vi "NF87XX.get channel.vi"(0 "i ref in":refnum<vi>, 2 "System":string, 5 "error in (no error)":errorcluster) -> (14 "i ref out":refnum<vi>, 16 "Channel":i32, 19 "error out":errorcluster)   [LabVIEW 2014, in "NF87XX.lvlib"]
doc: "Returns the actice motor channel if \"System\" is the name of one of the drivers, the driver is of type 1 (3-channel open loop driver), and the system answers without error. Otherwise 99999 is given out.\n\nauthor: Stefan Götte\ndata: 09-JAN-2007\n\n\nLicense Agreement for this software:\n\nCopyright (C)\nGesellschaft für Schwerionenforschung, GSI\nPlanckstr. 1\n64291 Darmstadt\nGermany\n\nContact: D.Beck@gsi.de \n\nThis program is free software; you can redistribute it and/or modify it under the terms of the GNU General Public License as published by the Free Software Foundation; either version 2 of the license, or (at your option) any later version.\n\nThis program is distributed in the hope that it will be useful, but WITHOUT ANY WARRANTY; without even the implied warranty of MERCHANTABILITY or FITNESS FOR A PARTICULAR PURPOSE. See the GNU General License for more details (http://www.gnu.org).\n\nGesellschaft für Schwerionenforschung, GSI\nPlanckstr. 1, 64291 Darmstadt, Germany\nFor all questions and ideas contact: M.Richter@gsi.de, H.Brand@gsi.de or D.Beck@gsi.de.\nLast update: 17-JUN-2004"
uses:
  NF87XX.lvlib
  instr.lib/NewFocusPico/Pico Parameters.ctl
  instr.lib/NewFocusPico/NewFocusPico - Driver np.lvlib
panel:
  in  "Pico Parameters":T1={"Pico Type"=enum."Open-Loop Pico", "Acceleration (steps/sec^2)"="32000", "Velocity ( Hz)"="2000", "Driver"="A1", "Motor"="0", "Channel"="0", "Process Step"="Final Test"}
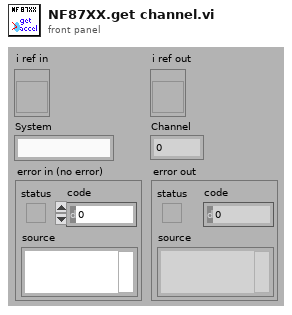
[diagram p1: front panel]
types:
  T1 = typedef "NewFocusPico - Driver np.lvlib/Pico Parameters.ctl" = cluster{"Pico Type":enum16{"Open-Loop Pico", "Close-Loop Pico", "Pico Ultra"}, "Acceleration (steps/sec^2)":string, "Velocity ( Hz)":string, "Driver":string, "Motor":string, "Channel":string, "Process Step":string}
  T2 = typedef "NF87XX.lvlib/NF87XX.driver Type.ctl" = enum16{"not defined", "3-ch open loop drv", "1-ch closed loop drv"}
  T3 = enum16{"User....", "DEF", "DIAG", "INI", "LOCK", "UNLOCK", "MAP", "SAV", "VER", "ACC", "CHL", "FOR", "GO", "HAL", "MOF", "MON", "MPV", "POS", "REL", "REV", "STA", "STO", "TYP", "VEL", "ABS", "SER", "NOS", "DRT", "FLI", "RLI", "FIN", "RIN", "AIN", "IN", "JOF", "JON", "OUT", "RES FINE", "RES COARSE", "02 (HEX)", "PWM", "CNT", "TMR", "HOSTNAME", "IPADDR", "IPMODE", "NETMASK", "GATEWAY", "DNSSRVR", "PASSWD", "ECHO", "MACADDR"}
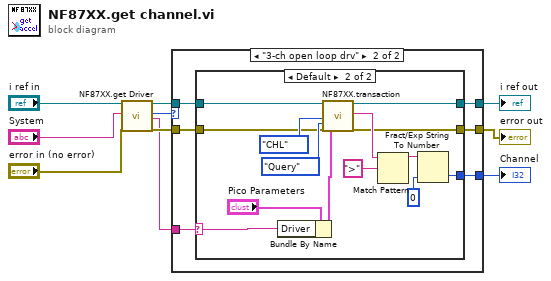
[diagram p0: block diagram]
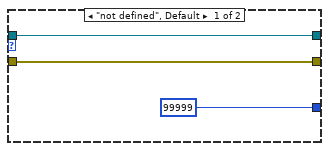
[diagram p2: hidden frame]
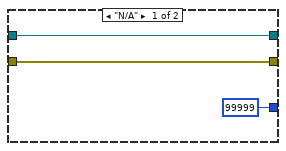
[diagram p3: hidden frame]
diagram:
  n1 = call "NF87XX.get Driver.vi"("i ref in"="i ref in", "System"="System", "error in (no error)"="error in (no error)") -> ("i ref out"=w4:refnum<vi>, "Driver Type"=w1:T2, "Driver"=w2:string, "error out"=w3:errorcluster)  [unwired: 12 in, 1 out]
  n2 = case shown="\"3-ch open loop drv\"" w1 {
    tunnel: [99999 w19] -> w10
    tunnel: [w13 w18] -> w9
    tunnel: [w12 w17] -> w8
    tunnel: w4 -> [w13 w16]
    tunnel: w3 -> [w12 w15]
    tunnel: w2 -> [_ w14]
    frame "not defined", Default {
    }
    frame "3-ch open loop drv" {
      n3 = case shown="Default" w14 {
        selector: w14 -> [_ w23]
        tunnel: [99999 w32] -> w19
        tunnel: [w22 w27] -> w18
        tunnel: [w21 w26] -> w17
        tunnel: w16 -> [w22 w25]
        tunnel: w15 -> [w21 w24]
        frame "N/A" {
        }
        frame Default {
          n4 = Bundle By Name(cluster="Pico Parameters", "Driver"=w23) -> (w30:T1)
          n5 = call "NF87XX.transaction.vi"("i ref in"=w25, "MCL Cmd"=T3."CHL", "Query/Set"=enum16{"Query", "Set"}."Query", "error in (no error)"=w24, "Pico Parameter"=w30) -> ("i ref out"=w27:refnum<vi>, "Read String"=w34:string, "error out"=w26:errorcluster)  [unwired: 12 in]
          n6 = Match Pattern(string=w34, regular expression=">" ("string")) -> (before substring=w28:string)  [unwired: 1 in, 3 out]
          n7 = Fract/Exp String To Number(string=w28, default (0 dbl)=0 ("default (0 DBL)")) -> (number=w32:i32)  [unwired: 2 in, 1 out]
        }
      }
    }
  }
  "error out" <- w8
  "i ref out" <- w9
  "Channel" <- w10
